vi "Threshold Color.vi"(2 "error in (no error)":errorcluster, 3 "Range":cluster{"Lower value":sgl, "Upper value":sgl}={"Lower value"=128.0, "Upper value"=255.0} {"Upper value" format="%.2f"; "Lower value" format="%.2f"}, 4 "Image Dst":T1, 5 "Image Src":T1) -> (0 "error out":errorcluster, 1 "Image Dst Out":T1)   [LabVIEW 2009, in "ImageProcessing.lvlib"]
doc: "Thresholds a grayscaled image and does som clean up"
uses:
  ImageProcessing.lvlib
  <vilib>/vision/Image Controls.llb/IMAQ Image.ctl
  <vilib>/vision/NI_Vision_Development_Module.lvlib
panel:
  out "Thresholded Image":T1(plugin-control) caption="HSL Threshold"
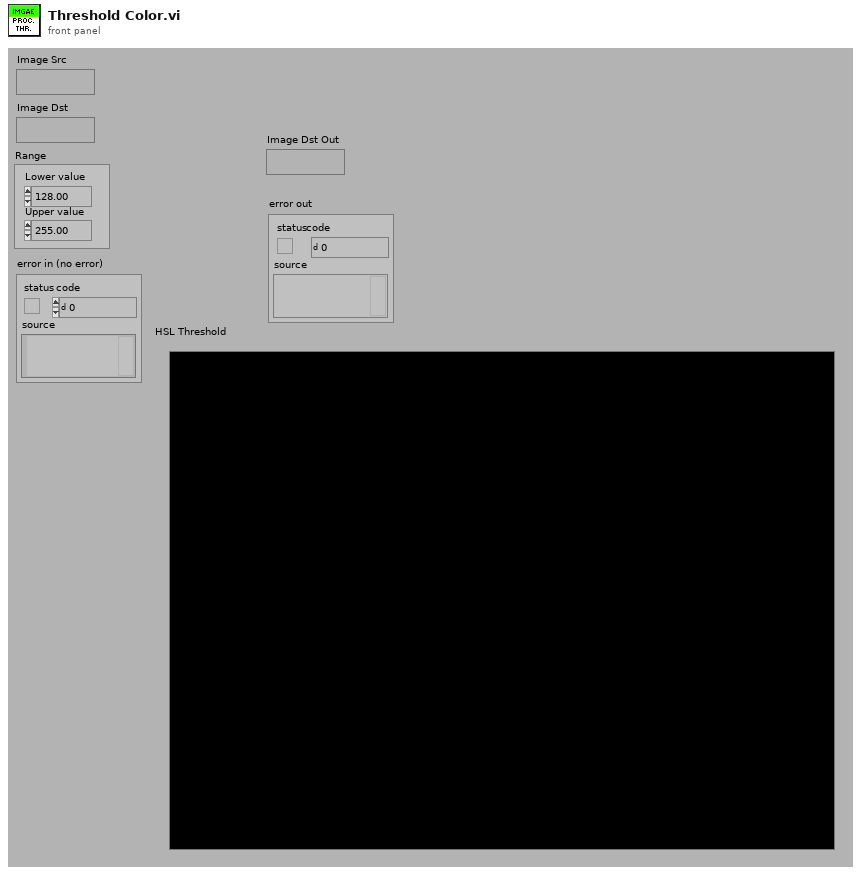
[diagram p1: front panel]
types:
  T1 = typedef "IMAQ Image.ctl" = refnum<image>
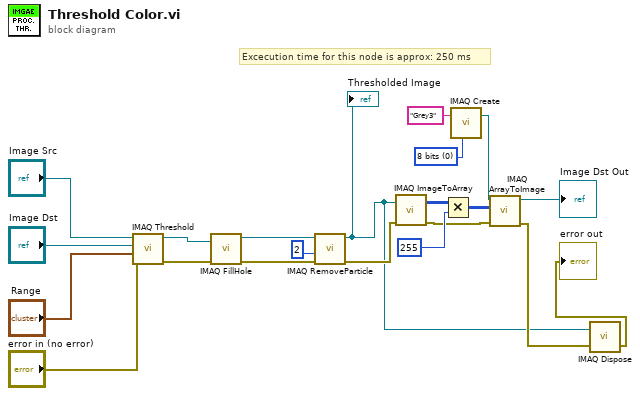
[diagram p0: block diagram]
diagram:
  w9 = u32 0 items=["8 bits", "16 bits", "Float", "Complex", "RGB", "HSL"] ("Image Type")
  # "Excecution time for this node is approx: 250 ms"
  n1 = call "IMAQ Threshold"("error in (no error)"="error in (no error)", "Range"="Range", "Image Dst"="Image Dst", "Image Src"="Image Src") -> ("error out"=w18:errorcluster, "Image Dst Out"=w6:T1)  [unwired: 6 in]
  n2 = call "IMAQ FillHole"("error in (no error)"=w18, "Image Src"=w6) -> ("error out"=w17:errorcluster, "Image Dst Out"=w14:T1)  [unwired: 2 in, 2 out]
  n3 = call "IMAQ RemoveParticle"("error in (no error)"=w17, "Number of Erosion"=2, "Image Src"=w14) -> ("error out"=w5:errorcluster, "Image Dst Out"=w1:T1)  [unwired: 4 in, 3 out]
  "Thresholded Image" <- w1
  n4 = call "IMAQ ImageToArray"("error in (no error)"=w5, "Image"=w1) -> ("error out"=w4:errorcluster, "Image Pixels (U8)"=w13:u8[][])  [unwired: 2 in, 3 out]
  n5 = Multiply(x=w13, y=255) -> (x*y=w11:i32[][])
  n6 = call "IMAQ Create"("Image Name"="Grey3", "Image Type"=w9) -> ("New Image"=w8:T1)  [unwired: 2 in, 2 out]
  n7 = call "IMAQ ArrayToImage"("error in (no error)"=w4, "Image Pixels (U8)"=w11, "Image"=w8) -> ("error out"=w3:errorcluster, "Image Out"=→"Image Dst Out":T1)  [unwired: 7 in]
  n8 = call "IMAQ Dispose"("Image"=w1, "error in (no error)"=w3) -> ("error out"=→"error out":errorcluster)  [unwired: 4 in]
